vi "potToDegrees.vi"(9 "POT VALUE AT 80*":dbl, 10 "POT VALUE AT 50*":dbl, 11 "POT VALUE":dbl) -> (3 "ANGLE":dbl)   [LabVIEW 2012]
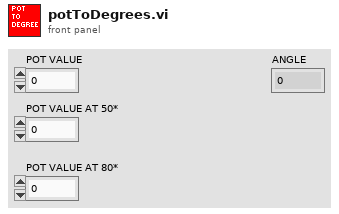
[diagram p1: front panel]
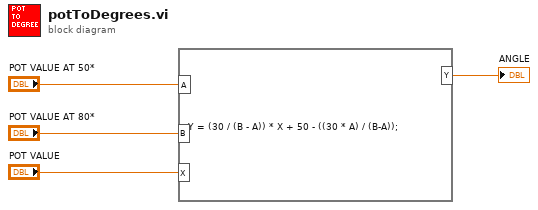
[diagram p0: block diagram]
diagram:
  n1 = formula code="Y = (30 / (B - A)) * X + 50 - ((30 * A) / (B-A));"("X"="POT VALUE", "B"="POT VALUE AT 80*", "A"="POT VALUE AT 50*") -> ("Y"=→"ANGLE":dbl)
